vi "Get Gas Refractive Index.vi"(1 "l (nm)":dbl, 2 "Gas":T1) -> (0 "n":cdb)   [LabVIEW 2015, in "Atmospheric Library.lvlib"]
doc: "Return the refractive index of the gas for the specified wavelength."
uses:
  Atmospheric Library.lvlib
  Gas.ctl
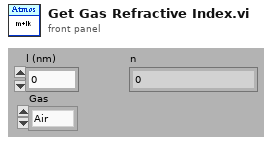
[diagram p1: front panel]
types:
  T1 = typedef "Atmospheric Library.lvlib/Gas.ctl" = enum16{"Air"}
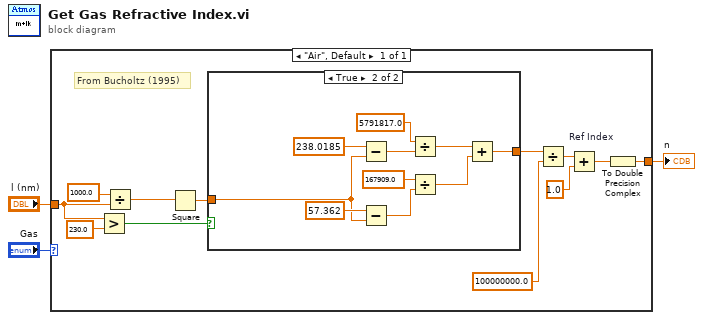
[diagram p0: block diagram]
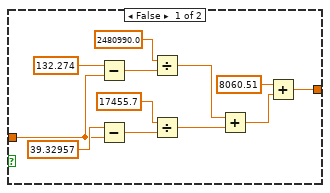
[diagram p2: hidden frame]
diagram:
  n1 = case shown="\"Air\", Default" "Gas" {
    tunnel: "l (nm)" -> [w8]
    tunnel: [w5] -> w2
    frame "Air", Default {
      # "From Bucholtz (1995)"
      n2 = Greater?(x=w8, y=230.0) -> (0:w6:bool)
      n3 = Divide(x=1000.0 ("y"), y=w8) -> (x/y=w10:dbl)
      n4 = Square(x=w10) -> (x^2=w9:dbl)
      n5 = case shown="True" w6 {
        tunnel: [w16 w37] -> w15
        tunnel: w9 -> [w19 w29]
        frame False {
          n6 = Subtract(x=132.274 ("y"), y=w19) -> (x-y=w26:dbl)
          n7 = Subtract(x=39.32957 ("y"), y=w19) -> (x-y=w23:dbl)
          n8 = Divide(x=2480990.0 ("y"), y=w26) -> (x/y=w24:dbl)
          n9 = Divide(x=17455.7 ("y"), y=w23) -> (x/y=w20:dbl)
          n10 = Add(x=w24, y=w20) -> (x+y=w18:dbl)
          n11 = Add(x=8060.51 ("y"), y=w18) -> (x+y=w16:dbl)
        }
        frame True {
          n12 = Subtract(x=238.0185 ("y"), y=w29) -> (x-y=w35:dbl)
          n13 = Subtract(x=57.362 ("y"), y=w29) -> (x-y=w32:dbl)
          n14 = Divide(x=5791817.0 ("y"), y=w35) -> (x/y=w33:dbl)
          n15 = Divide(x=167909.0 ("y"), y=w32) -> (x/y=w28:dbl)
          n16 = Add(x=w33, y=w28) -> (x+y=w37:dbl)
        }
      }
      n17 = Divide(x=w15, y=100000000.0) -> (x/y=w13:dbl)
      n18 = Add "Ref Index"(x=w13, y=1.0) -> (x+y=w4:dbl)
      n19 = To Double Precision Complex(1:w4) -> (0:w5:cdb)
    }
  }
  "n" <- w2
